vi "Example.vi"() -> ()   [LabVIEW 2019, in "Valve1DO1DI.lvclass"]
uses:
  Valve1DO1DI.lvclass
  D:/GIT H4000/H4000/src/Proccess_class/Proccess.lvclass
  ConfigJSON_class/ConfigJSON.lvclass
  D:/GIT H4000/H4000/src/ConfigInterface_class/ConfigInterface.lvclass
  MessageAMC_class/MessageAMC.lvclass
  D:/GIT H4000/H4000/src/MessageInterface_class/MessageInterface.lvclass
  Logger_class/Logger.lvclass
  <vilib>/NI/AMC/AMC.lvlib
  Proccess_class/Proccess.lvclass
panel:
  in  "stop":bool
  out "error out":errorcluster
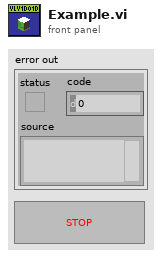
[diagram p1: front panel]
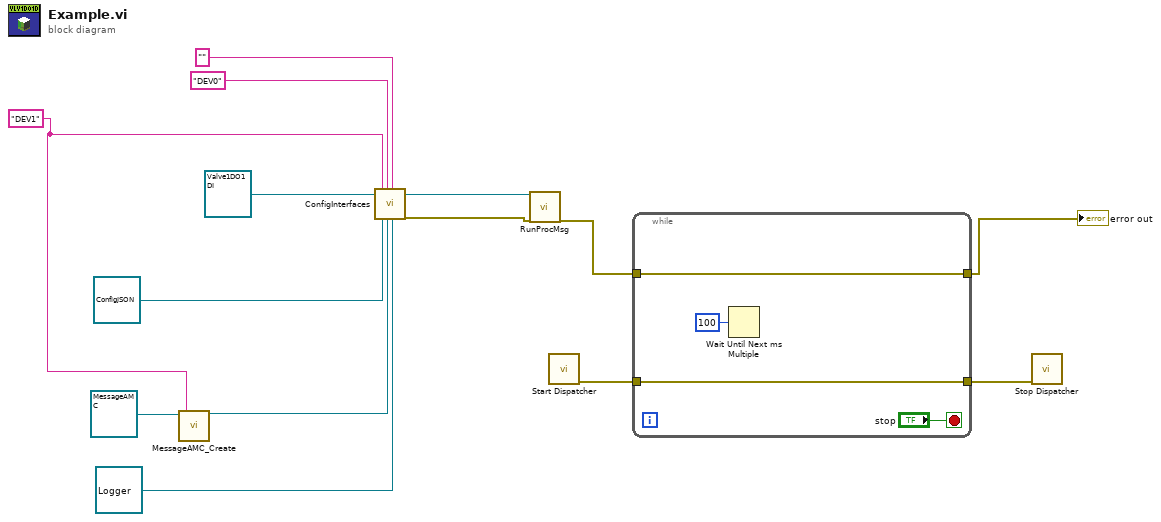
[diagram p0: block diagram]
diagram:
  w1 = "DEV1" ("Name")
  n1 = call "MessageAMC_Create.vi"("reference in"=refnum<class "MessageAMC.lvclass"> refnum ("MessageAMC"), "message queue name"=w1) -> ("amc"=w7:refnum<class "MessageAMC.lvclass">)  [unwired: 16 in, 1 out]
  n2 = call "ConfigInterfaces.vi"("reference in"=refnum<class "Valve1DO1DI.lvclass"> refnum, "Name"=w1, "ConfigInterface"=refnum<class "ConfigJSON.lvclass"> refnum ("ConfigJSON"), "ParentName"="DEV0", "MessageInterface"=w7, "Description"="" ("desc"), "Logger"=refnum<class "Logger.lvclass"> refnum) -> ("reference out"=w4:refnum<class "Valve1DO1DI.lvclass">, "error out"=w5:errorcluster)  [unwired: 11 in]
  n3 = call-dynamic "RunProcMsg.vi"("reference in"=w4, "error in (no error)"=w5) -> ("error out"=w13:errorcluster)  [unwired: 16 in, 1 out]
  n4 = call <vilib>:"Start Dispatcher.vi"() -> ("error out"=w10:errorcluster)  [unwired: 13 in, 2 out]
  n5 = while {
    tunnel: w13 -> [w18]
    tunnel: [w18] -> w12
    tunnel: [w15] -> w11
    tunnel: w10 -> [w15]
    stop <- "stop" stop-if-true
    n6 = Wait Until Next ms Multiple(millisecond multiple=u32 100) -> ()  [unwired: 1 out]
  }
  "error out" <- w12
  n7 = call <vilib>:"Stop Dispatcher.vi"("error in"=w11) -> ()  [unwired: 14 in, 1 out]
